vi "Get Environment.vi"(8 "error in":errorcluster, 10 "?":T1, 11 "Paths":T2) -> (0 "error out":errorcluster, 3 "Environment out":refnum<k24>)   [LabVIEW 2024, in "WebView.lvclass"]
uses:
  <vilib>/sklein/WebView2/Libs/Microsoft.Web.WebView2.Core.dll
  WebView.lvclass
  WebView.lvclass/WebView.ctl
  Paths-cluster.ctl
  Core Envrionment Options--cluster.ctl
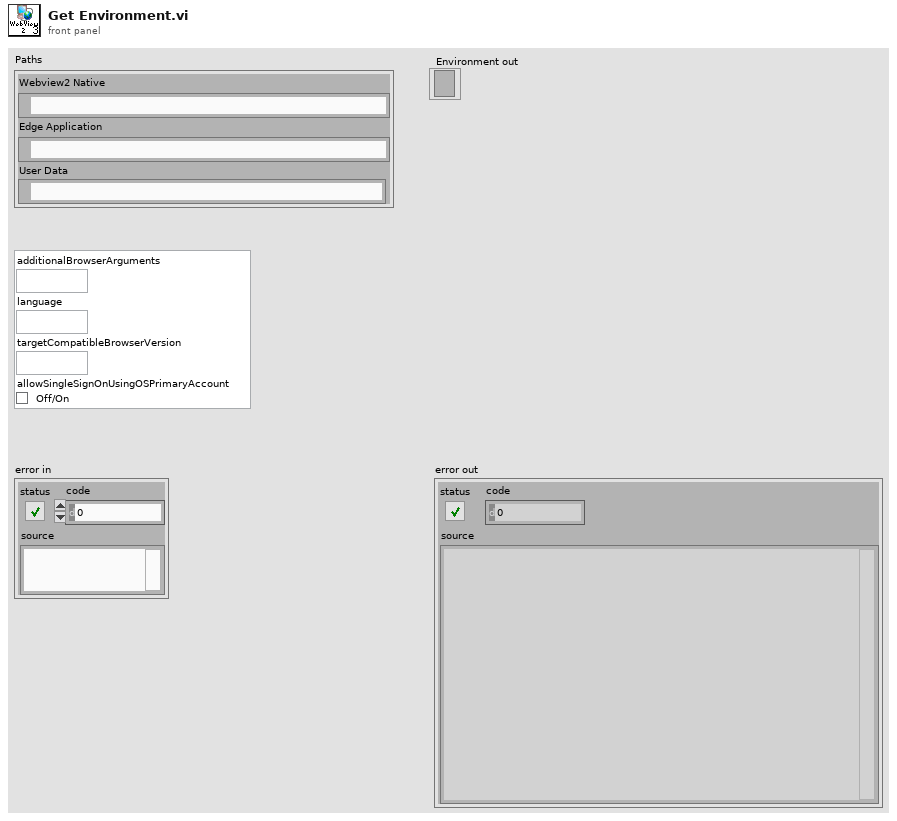
[diagram p1: front panel]
types:
  T1 = typedef "Core Envrionment Options--cluster.ctl" = cluster{"additionalBrowserArguments":string, "language":string, "targetCompatibleBrowserVersion":string, "allowSingleSignOnUsingOSPrimaryAccount":bool}
  T2 = typedef "WebView.lvclass/Paths-cluster.ctl" = cluster{"Webview2 Native":path, "Edge Application":path, "User Data":path}
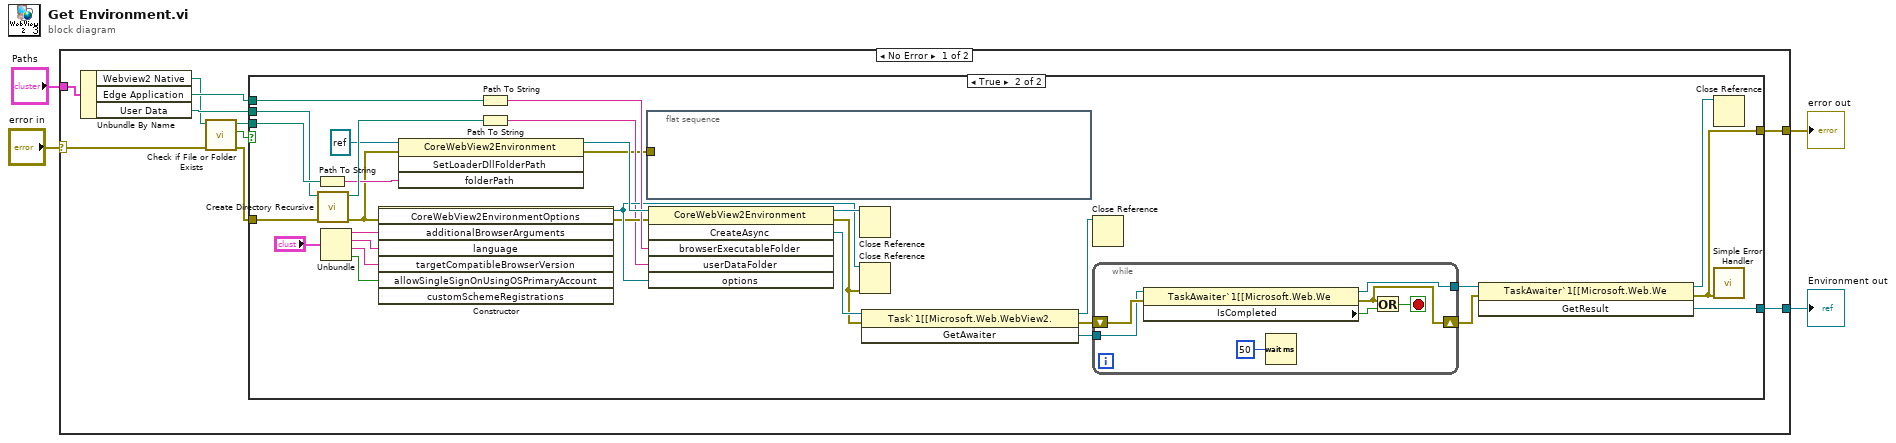
[diagram p0: block diagram]
diagram:
  n1 = case shown="No Error" "error in" {
    selector: "error in" -> [w11 w53]
    tunnel: [w14 w53] -> w4
    tunnel: [w13 _] -> w3
    tunnel: "Paths" -> [w12 _]
    frame No Error {
      n2 = Unbundle By Name(w12) -> ("Webview2 Native"=w7:path, "Edge Application"=w10:path, "User Data"=w9:path)
      n3 = call <vilib>:"Check if File or Folder Exists.vi"("error in (no error)"=w11, "path"=w7) -> ("error out"=w8:errorcluster, "file or folder exists?"=w5:bool, "dup path"=w6:path)  [unwired: 7 in]
      n4 = case shown="True" w5 {
        tunnel: w10 -> [_ w42]
        tunnel: w9 -> [_ w36]
        tunnel: [_ w16] -> w13
        tunnel: [w15 w32] -> w14
        tunnel: w8 -> [w15 w37]
        tunnel: w6 -> [_ w38]
        frame False {
        }
        frame True {
          n5 = Path To String(path=w38) -> (string=w21:string)
          n6 = call <vilib>:"Create Directory Recursive.vi"("error in (no error)"=w37, "directory"=w36) -> ("error out"=w19:errorcluster, "directory copy"=w24:path)  [unwired: 3 in, 1 out]
          n7 = Unbundle("?") -> ("additionalBrowserArguments"=w30:string, "language"=w29:string, "targetCompatibleBrowserVersion"=w28:string, "allowSingleSignOnUsingOSPrimaryAccount"=w27:bool)
          n8 = constructor class="CoreWebView2EnvironmentOptions"(error in=w19, "additionalBrowserArguments"=w30, "language"=w29, "targetCompatibleBrowserVersion"=w28, "allowSingleSignOnUsingOSPrimaryAccount"=w27) -> (reference out=w26:refnum<k24>, error out=w25:errorcluster)  [unwired: 3 in, 6 out]
          n9 = invoke class="CoreWebView2Environment" method="SetLoaderDllFolderPath"(reference=refnum<k24> refnum ("environment"), error in=w19, "folderPath"=w21) -> (reference out=w45:refnum<k24>, error out=w20:errorcluster)  [unwired: 1 in, 2 out]
          n10 = Path To String(path=w42) -> (string=w44:string)
          n11 = Path To String(path=w24) -> (string=w23:string)
          n12 = flat-sequence {
            tunnel: w20 -> [_]
            frame #0 {
            }
          }
          n13 = invoke class="CoreWebView2Environment" method="CreateAsync"(reference=w45, error in=w25, "browserExecutableFolder"=w44, "userDataFolder"=w23, "options"=w26) -> (reference out=w34:refnum<k24>, error out=w17:errorcluster, "CreateAsync"=w43:refnum<k24>)  [unwired: 1 in, 3 out]
          n14 = Close Reference(reference=w34) -> ()  [unwired: 1 in, 1 out]
          n15 = Close Reference(reference=w26, error in (no error)=w17) -> ()  [unwired: 1 out]
          n16 = invoke class="Task`1[[Microsoft.Web.WebView2." method="GetAwaiter"(reference=w43, error in=w17) -> (reference out=w39:refnum<k24>, error out=w41:errorcluster, "GetAwaiter"=w18:refnum<k24>)  [unwired: 1 in]
          n17 = Close Reference(reference=w39) -> ()  [unwired: 1 in, 1 out]
          n18 = while {
            tunnel: w18 -> [w51]
            shift-right: [w46] -> w33
            shift-left: w41 -> [w52]
            tunnel: [w48] -> w40
            stop <- w47 stop-if-true
            n19 = property class="TaskAwaiter`1[[Microsoft.Web.We"(reference=w51, error in=w52) -> (reference out=w48:refnum<k24>, error out=w46:errorcluster, "IsCompleted"=w49:bool)
            n20 = Wait (ms)(milliseconds to wait=u32 50 ("millisecond multiple")) -> ()  [unwired: 1 out]
            n21 = Or(x=w46, y=w49) -> (x .or. y?=w47:bool)
          }
          n22 = invoke class="TaskAwaiter`1[[Microsoft.Web.We" method="GetResult"(reference=w40, error in=w33) -> (reference out=w35:refnum<k24>, error out=w32:errorcluster, "GetResult"=w16:refnum<k24>)  [unwired: 1 in]
          n23 = Close Reference(reference=w35) -> ()  [unwired: 1 in, 1 out]
          n24 = call <vilib>:"Simple Error Handler.vi"("error in (no error)"=w32) -> ()  [unwired: 4 in, 5 out]
        }
      }
    }
    frame Error {
    }
  }
  "error out" <- w4
  "Environment out" <- w3
